vi "WVDIAL Initiate Pulses.vi"() -> ()   [LabVIEW 2012]
doc: "This VI is an example of how to use subVIs from the QC 9000 series driver to programmatically configure multiple channels and the system timer (To). This VI initializes the pulse generator, gets the number of channels in the unit, configures individual channel(s), configures the system timer (To), initiate pulse generation, and then closes communications with the pulse generator. By default the VI DOES NOT stop pulse generation when exiting!!! Not all trigger and gate features are supported by all models covered by this driver. Selection of an unsupported function will generate a software error and the command is not sent to the hardware.\n\n\nNotes:\n1) The pulse generator keypad is returned to \"Local\" mode when this VI terminates in order to restore manual control to the user.\n2) VISA Version 3.3 or higher must be installed to use this instrument driver."
uses:
  Support/Channel Parameters.ctl
  Support/System Parameters.ctl
  Berkeley Nucleonics 500 Series.lvlib
panel:
  in  "VISA resource":refnum<visa-resource-name>="Berkeley_PG"
  in  "System Paramaters":T1={"Sys Period"=0.000142, "Sys Mode"=enum."Normal", "Sys Burst #"=0, "Sys DC On"=10, "Sys DC Off"=20, "Sys State"=FALSE, "Sys Gate"=TRUE, "Sys Trig Edge"=TRUE, "Sys Ext Mode"=enum."Disabled", "Sys Trig Lev"=2.5, "Sys Gate Lev "=2.5, "Sys Gate Mode"=enum."Disabled"} {"Sys Gate Lev" format="%.4p"; "Sys Trig Lev" format="%.4p"; "Sys Period" format="%.6p"}
  in  "Channel Parameters":T2[](array[typedef])=[{"Channel"=1, "Chan State"=TRUE, "Chan Sync Source"=0, "Chan Gate Logic"=enum."High", "Chan Mode"=enum."Normal", "Chan Wait #"=0, "Chan Delay"=1e-07, "Chan Width"=1e-06, "Chan Burst #"=0, "Chan DC On"=0, "Chan DC Off"=0, "Chan Polarity"=FALSE, "Chan MUX Value"=-1, "Chan Level Out"=enum."TTL", "Chan Lev Adjust"=0.0, "Chan Gate Mode"=enum."Disabled"}, {"Channel"=1, "Chan State"=TRUE, "Chan Sync Source"=0, "Chan Gate Logic"=enum."High", "Chan Mode"=enum."Normal", "Chan Wait #"=0, "Chan Delay"=1e-07, "Chan Width"=1e-06, "Chan Burst #"=0, "Chan DC On"=0, "Chan DC Off"=0, "Chan Polarity"=FALSE, "Chan MUX Value"=-1, "Chan Level Out"=enum."TTL", "Chan Lev Adjust"=0.0, "Chan Gate Mode"=enum."Disabled"}, {"Channel"=2, "Chan State"=TRUE, "Chan Sync Source"=0, "Chan Gate Logic"=enum."High", "Chan Mode"=enum."Normal", "Chan Wait #"=1, "Chan Delay"=1e-07, "Chan Width"=1e-06, "Chan Burst #"=0, "Chan DC On"=0, "Chan DC Off"=0, "Chan Polarity"=FALSE, "Chan MUX Value"=-1, "Chan Level Out"=enum."TTL", "Chan Lev Adjust"=0.0, "Chan Gate Mode"=enum."Disabled"}, {"Channel"=3, "Chan State"=TRUE, "Chan Sync Source"=0, "Chan Gate Logic"=enum."High", "Chan Mode"=enum."Duty Cycle", "Chan Wait #"=0, "Chan Delay"=1e-07, "Chan Width"=0.00994, "Chan Burst #"=0, "Chan DC On"=1, "Chan DC Off"=139, "Chan Polarity"=FALSE, "Chan MUX Value"=-1, "Chan Level Out"=enum."TTL", "Chan Lev Adjust"=0.0, "Chan Gate Mode"=enum."Disabled"}, {"Channel"=4, "Chan State"=TRUE, "Chan Sync Source"=0, "Chan Gate Logic"=enum."High", "Chan Mode"=enum."Duty Cycle", "Chan Wait #"=0, "Chan Delay"=1e-07, "Chan Width"=0.00994, "Chan Burst #"=0, "Chan DC On"=1, "Chan DC Off"=139, "Chan Polarity"=FALSE, "Chan MUX Value"=-1, "Chan Level Out"=enum."TTL", "Chan Lev Adjust"=0.0, "Chan Gate Mode"=enum."Disabled"}, {"Channel"=5, "Chan State"=TRUE, "Chan Sync Source"=0, "Chan Gate Logic"=enum."High", "Chan Mode"=enum."Duty Cycle", "Chan Wait #"=70, "Chan Delay"=1e-07, "Chan Width"=0.00994, "Chan Burst #"=0, "Chan DC On"=1, "Chan DC Off"=139, "Chan Polarity"=FALSE, "Chan MUX Value"=-1, "Chan Level Out"=enum."TTL", "Chan Lev Adjust"=0.0, "Chan Gate Mode"=enum."Disabled"}, {"Channel"=6, "Chan State"=TRUE, "Chan Sync Source"=0, "Chan Gate Logic"=enum."Low", "Chan Mode"=enum."Duty Cycle", "Chan Wait #"=0, "Chan Delay"=0.0, "Chan Width"=1.1e-06, "Chan Burst #"=0, "Chan DC On"=70, "Chan DC Off"=70, "Chan Polarity"=FALSE, "Chan MUX Value"=-1, "Chan Level Out"=enum."TTL", "Chan Lev Adjust"=0.0, "Chan Gate Mode"=enum."Disabled"}, {"Channel"=7, "Chan State"=TRUE, "Chan Sync Source"=0, "Chan Gate Logic"=enum."Low", "Chan Mode"=enum."Duty Cycle", "Chan Wait #"=70, "Chan Delay"=0.0, "Chan Width"=1.1e-06, "Chan Burst #"=0, "Chan DC On"=70, "Chan DC Off"=70, "Chan Polarity"=FALSE, "Chan MUX Value"=-1, "Chan Level Out"=enum."TTL", "Chan Lev Adjust"=0.0, "Chan Gate Mode"=enum."Disabled"}, {"Channel"=8, "Chan State"=TRUE, "Chan Sync Source"=0, "Chan Gate Logic"=enum."High", "Chan Mode"=enum."Normal", "Chan Wait #"=0, "Chan Delay"=0.0, "Chan Width"=1e-06, "Chan Burst #"=0, "Chan DC On"=0, "Chan DC Off"=0, "Chan Polarity"=FALSE, "Chan MUX Value"=-1, "Chan Level Out"=enum."TTL", "Chan Lev Adjust"=0.0, "Chan Gate Mode"=enum."Disabled"}] {"Chan Sync Source" items=["System (To)", "Channel A", "Channel B", "Channel C", "Channel D", "Channel E", "Channel F", "Channel G", "Channel H"]; "Chan Width" format="%.3p"; "Chan Delay" format="%.3p"; "Chan Lev Adjust" format="%.3p"; "Channel" items=["Channel A"=1, "Channel B"=2, "Channel C"=3, "Channel D"=4, "Channel E"=5, "Channel F"=6, "Channel G"=7, "Channel H"=8]}
  # "500 Series\nPulse Generator\nExample Program"
  # "NOTES: Make sure instrument baud rate is \nset to the same value as in the initialize.vi"
  # "Notes:\n1.  The channel parameters \"Burst #\", \"DC On\", \"DC Off\", and \"Adjustable\" are only updated when operating in the corresponding mode.\n2.  The system parameters  \"Burst #\", \"DC On\", \"DC Off\", and \"Trig Level\"` are only updated when operating in the corresponding mode."
  # "Input"
  # "Triggered"
  # "Gated"
  # "Mode"
  # "Burst"
  # "Duty\nCycle"
  # "Input"
  # "Normal\nSingle\nBurst"
  # "Burst"
  # "Duty Cycle"
  # "Output"
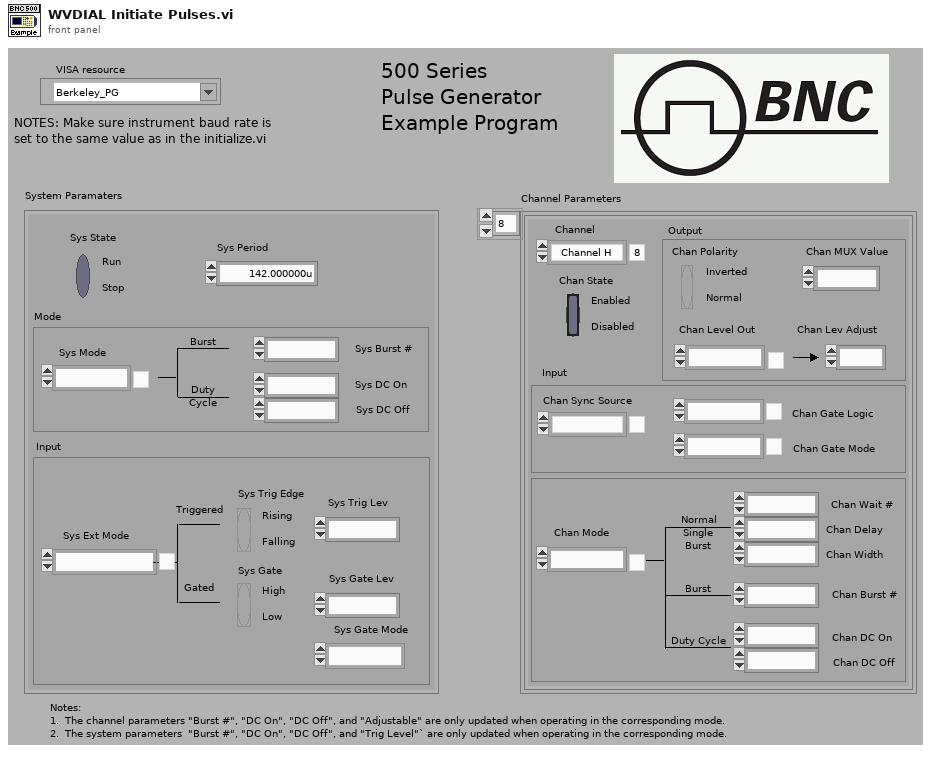
[diagram p1: front panel]
types:
  T1 = typedef "System Parameters.ctl" = cluster{"Sys Period":dbl, "Sys Mode":enum16{"Normal", "Single", "Burst", "Duty Cycle"}, "Sys Burst #":i32, "Sys DC On":i32, "Sys DC Off":i32, "Sys State":bool, "Sys Gate":bool, "Sys Trig Edge":bool, "Sys Ext Mode":enum16{"Disabled", "Triggered", "Gated", "Triggered & Gated"}, "Sys Trig Lev":dbl, "Sys Gate Lev ":dbl, "Sys Gate Mode":enum16{"Disabled", "Pulse Inhibit", "Output Inhibit", "Channel"}}
  T2 = typedef "Channel Parameters.ctl" = cluster{"Channel":i32, "Chan State":bool, "Chan Sync Source":i32, "Chan Gate Logic":enum16{"Disabled", "Low", "High"}, "Chan Mode":enum16{"Normal", "Single", "Burst", "Duty Cycle"}, "Chan Wait #":i32, "Chan Delay":dbl, "Chan Width":dbl, "Chan Burst #":i32, "Chan DC On":i32, "Chan DC Off":i32, "Chan Polarity":bool, "Chan MUX Value":i32, "Chan Level Out":enum16{"TTL", "Adjustable", "35 Volt", "Optical"}, "Chan Lev Adjust":dbl, "Chan Gate Mode":enum16{"Disabled", "Pulse Inhibit", "Output Inhibit"}}
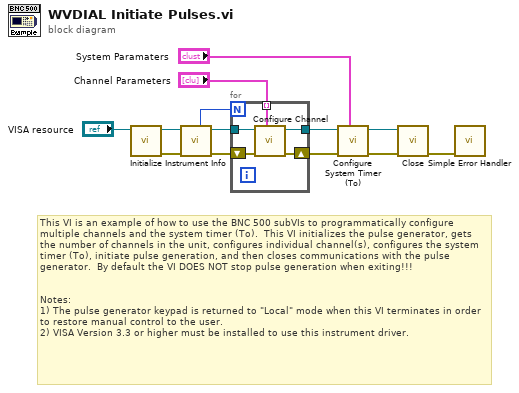
[diagram p0: block diagram]
diagram:
  # "This VI is an example of how to use the BNC 500 subVIs to programmatically configure multiple channels and the system timer (To).  This VI initializes the pulse generator, gets the number of channels in the unit, configures individual channel(s), configures the system timer (To), initiate pulse generation, and then closes communications with the pulse generator.  By default the VI DOES NOT stop pulse generation when exiting!!!\n\n\nNotes:\n1) The pulse generator keypad is returned to \"Local\" mode when this VI terminates in order to restore manual control to the user.\n2) VISA Version 3.3 or higher must be installed to use this instrument driver."
  n1 = call "Initialize.vi"("VISA resource name"="VISA resource") -> ("error out"=w5:errorcluster, "VISA resource name out"=w6:refnum<visa-resource-name>)  [unwired: 4 in, 5 out]
  n2 = call "Instrument Info.vi"("error in (no error)"=w5, "VISA resource name"=w6) -> ("error out"=w3:errorcluster, "VISA resource name out"=w7:refnum<visa-resource-name>, "Channels"=w2:i32)  [unwired: 7 out]
  n3 = for {
    N: w2 -> [_]
    tunnel: [w18] -> w13
    tunnel: "Channel Parameters" -> [w17] mode=indexing
    tunnel: w7 -> [w16]
    shift-right: [w15] -> w4
    shift-left: w3 -> [w14]
    n4 = call "Configure Channel.vi"("Chan Parameters"=w17, "error in (no error)"=w14, "VISA resource name"=w16) -> ("error out"=w15:errorcluster, "VISA resource name out"=w18:refnum<visa-resource-name>)  [unwired: 7 out]
  }
  n5 = call "Configure System Timer (To).vi"("System Parameters"="System Paramaters", "error in (no error)"=w4, "VISA resource name"=w13) -> ("error out"=w8:errorcluster, "VISA resource name out"=w9:refnum<visa-resource-name>)  [unwired: 7 out]
  n6 = call "Close.vi"("error in (no error)"=w8, "VISA resource name"=w9) -> ("error out"=w1:errorcluster)  [unwired: 9 out]
  n7 = call <vilib>:"Simple Error Handler.vi"("error in (no error)"=w1) -> ()  [unwired: 1 in, 8 out]
